vi "VEL.vi"(0 "System no.":i32=1 min=1 max=4 step=1, 2 "Axes to set":string[](array[string]), 3 "Velocity values":dbl[](array[numeric]) format="%.6f", 4 "No.of digits":i16=4, 5 "error in":errorcluster, 6 "Without axis ID?":bool) -> (14 "Controller error":bool, 19 "error out":errorcluster)   [LabVIEW 2026]
doc: "Sets velocity and checks for error. If Without axis ID? is TRUE, then Axes to set is ignored and first field of Velocity values array is used for velocity command. The velocity should not be set to 0. Number of digits is the number of digits after the decimal point in the velocity value(s) that will be sent. Controller error is TRUE if selected system reports an error code which is not 0.\n\nAnalog: Without axis ID? = FALSE; Velocity unit is µm/sec\n\nC-413: Without axis ID? = FALSE. Velocity unit is mm/s. Velocity settings made with VEL are present in RAM only and will be reset to default (parameter 0x06010400) when the controller is powered down or rebooted.\n\nC-867, C-877, C-884, C-891, Hydra, Pollux, Mercury_GCS: Without axis ID? = FALSE. Velocity unit is mm/s. The VEL command saves the parameters in RAM only. To save the currently valid parameters to flash ROM, where they become the power-on defaults, you must run WPA.vi. Parameter changes not saved with WPA will be lost when the controller is powered off.\n\nC-880: Without axis ID? = FALSE, for NanoCube axes command is not valid\n\nC-880K005: VI only supported when called through PI_Multix.vi\n\nC-885: Without axis ID? = FALSE. The VEL command saves the parameters in RAM only. For how to save the currently valid parameters to flash ROM, where they become the power-on defaults, please refer to the controller's user manual.\n\nE-516: Without axis ID? = FALSE. Velocity unit is µm/s. The VEL command saves the parameters in RAM only. To save the currently valid parameters to flash ROM, where they become the power-on defaults, you must run WPA.vi. Parameter changes not saved with WPA will be lost when the E-516 is powered off.\n\nE -517, E-518: Without axis ID? = FALSE. Velocity unit is µm/s in closed-loop operation and V/s in open-loop operation. Velocity settings made with VEL are present in RAM only and will be reset to default (\"Servo Loop Slew Rate\" value) when the controller is powered down or rebooted.\n\nE-709, E-712, E-725, E-727, E-753, E-754, E-861: Without axis ID? = FALSE. Velocity unit is µm/s. Velocity settings made with VEL are present in RAM only and will be reset to default (\"Servo Loop Slew Rate\" value) when the controller is powered down or rebooted.\n\nE-710: Without axis ID? = FALSE. Velocity unit is µm/ms.\n\nE-755: Without axis ID? = FALSE. Velocity unit is µm/s. Command not available for E-755.101.\n\nE-761: Without axis ID? = FALSE. Velocity unit is µm/ms.The VEL command saves the \"Servo Loop Slew Rate\" parameter in RAM only. To save the currently valid parameter to flash ROM, where it becomes the power-on defaults, you must run WPA.vi. Parameter changes not saved with WPA will be lost when the PC is powered off or the E-761 is rebooted.\n\nE-861: Without axis ID? = FALSE. The VEL setting only takes effect when the given axis is in closed-loop operation (servo on). For open-loop operation, use OVL instead. The maximum value which can be set with the VEL command is given by the Closed-loop velocity parameter, ID 0xA (can be changed with SPA and SEP). On power-on, the current closed-loop velocity is half the maximum.\n\nE-873, E-874: Without axis ID? = FALSE. The VEL command saves the parameters in RAM only. To save the currently valid parameters to flash ROM, where they become the power-on defaults, you must run WPA.vi. Parameter changes not saved with WPA will be lost when the controller is powered off.\n\nC-886: VEL command is only valid for velocity of additional axes. To set velocity of the parallel kinematics, please use the VLS command instead.\n\nC-887, F-206, M-8X0: For GCS syntax version = GCS 2.0 or higher (Check with CSV?.vi. If CSV?.vi is not supported, syntax version is GCS 1.0), VEL command is only valid for velocity of axes A and/or B, Without axis ID? = False. For platform velocity, VI sends command VLS instead, in this case Without axis ID? = TRUE. For axes K, L, M command is not valid.\nFor GCS syntax version = GCS 1.0, to set platform velocity: Without axis ID? = TRUE; to set velocity of axes A and/or B: Without axis ID? = False; axes K, L, M: command not valid. \n\nAll other systems: Without axis ID? = FALSE"
uses:
  Controller names.ctl
  Communication/Syntax.ctl
  Communication/Global1.vi
  Global2 (Array).vi
panel:
  # "Sets velocity and checks for error.  If \"Without axis ID\" is TRUE, \nthen \"Axes to set\" is ignored and first field of \"Velocity values\" \narray is used for velocity command by sending VEL for GCS 1.0 \nand VLS for GCS 2.0 or higher."
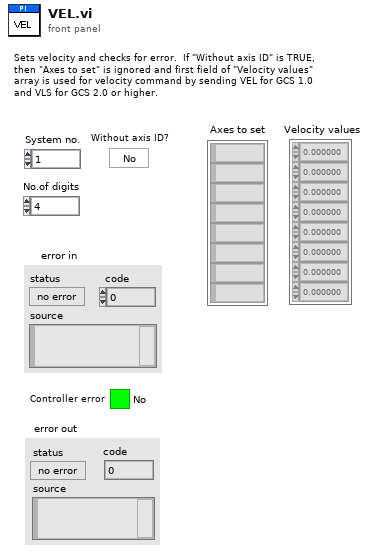
[diagram p1: front panel]
types:
  T1 = typedef "Syntax.ctl" = enum16{"GCS 1.0", "GCS 2.0", "GCS 3.0"}
  T2 = enum16{"Disable error check", "Force error check", "Use global settings"}
  T3 = typedef "Controller names.ctl" = enum16{"None", "Analog", "C-702", "C-413", "C-414", "C-843", "C-843.PM", "C-844", "C-848", "C-865", "C-866", "C-867", "C-877", "C-880", "C-884", "C-885", "C-886", "C-887", "C-891", "E-135", "E-516", "E-517", "E-518", "E-709", "E-710", "E-712", "E-725", "E-727", "E-753", "E-754", "E-755", "E-761", "E-816", "E-861", "E-870", "E-871", "E-872", "E-873", "E-874", "F-206", "HydraPollux", "M-840", "M-850", "M-8X0", "Mercury", "Mercury_GCS", "PI_GCS2"}
  T4 = cluster{"Conn. axes":string[], "Controller name":T3}[]
  T5 = cluster{"Conn. axes":string[], "Controller name":T3}
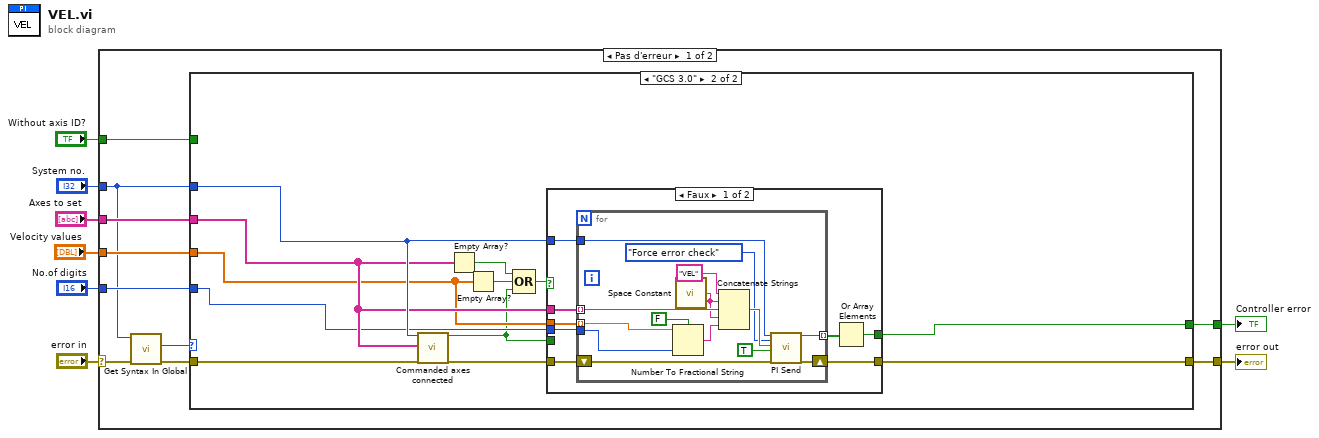
[diagram p0: block diagram]
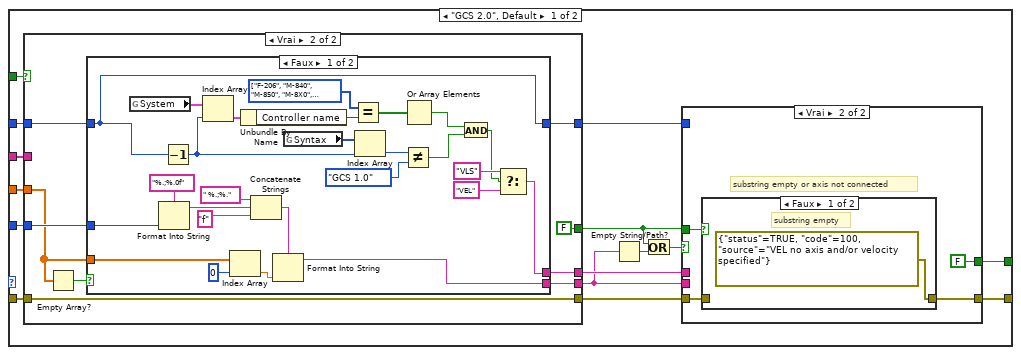
[diagram p2: hidden frame]
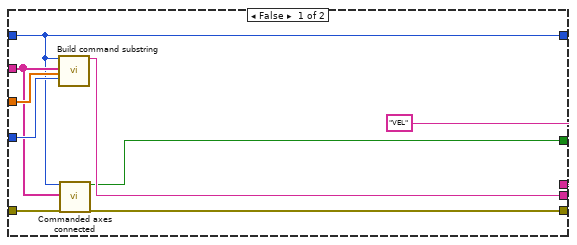
[diagram p3: hidden frame]
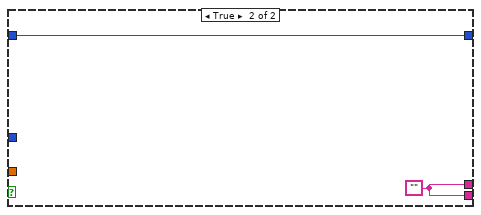
[diagram p4: hidden frame]
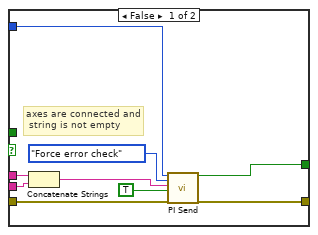
[diagram p5: hidden frame]
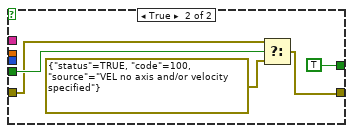
[diagram p7: hidden frame]
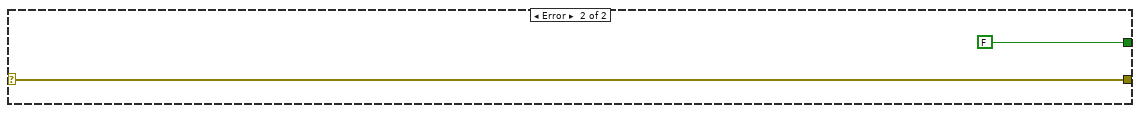
[diagram p8: hidden frame]
diagram:
  n1 = case shown="Pas d'erreur" "error in" {
    selector: "error in" -> [w11 w135]
    tunnel: [w18 w135] -> w8
    tunnel: "Velocity values" -> [w17 _]
    tunnel: "No.of digits" -> [w16 _]
    tunnel: "System no." -> [w9 _]
    tunnel: "Axes to set" -> [w15 _]
    tunnel: "Without axis ID?" -> [w14 _]
    tunnel: [w13 FALSE ("Controller error")] -> w1
    frame No Error {
      n2 = call "Get Syntax In Global.vi"("error in"=w11, "System no."=w9) -> ("error out"=w10:errorcluster, "Syntax"=w12:T1)  [unwired: 8 in]
      n3 = case shown="\"GCS 3.0\"" w12 {
        tunnel: [w33 w105] -> w18
        tunnel: w17 -> [w32 w101]
        tunnel: w16 -> [w31 w100]
        tunnel: w15 -> [w29 w102]
        tunnel: w14 -> [w28 _]
        tunnel: w9 -> [w27 w103]
        tunnel: w10 -> [w25 w104]
        tunnel: [w19 w96] -> w13
        frame "GCS 2.0", Default {
          n4 = case shown="Vrai" w28 {
            tunnel: [w42 w49] -> w24
            tunnel: w32 -> [w41 w46]
            tunnel: w31 -> [w40 w48]
            tunnel: w25 -> [w39 w51]
            tunnel: [w38 w51] -> w30
            tunnel: w29 -> [w37 _]
            tunnel: [w36 FALSE] -> w22
            tunnel: w27 -> [w34 w44]
            tunnel: ["VEL" w47] -> w26
            tunnel: [w34 w43] -> w20
            frame False {
              n5 = call "Build command substring.vi"("System no."=w34, "Affected axes"=w37, "Parameters"=w41, "No. of digits"=w40) -> ("Command substring"=w42:string)  [unwired: 3 in, 12 out]
              n6 = call "Commanded axes connected.vi"("System no."=w34, "Commanded axes"=w37, "error in"=w39) -> ("Controller error"=w36:bool, "error out"=w38:errorcluster)  [unwired: 1 in, 14 out]
            }
            frame True {
              n7 = Empty Array?(array=w46) -> (empty?=w45:bool)
              n8 = case shown="Faux" w45 {
                tunnel: [w77 w79] -> w49
                tunnel: w48 -> [w72 _]
                tunnel: w46 -> [w70 _]
                tunnel: [w56 w79] -> w47
                tunnel: w44 -> [w52 w78]
                tunnel: [w52 w78] -> w43
                frame False {
                  w66 = T3[] [enum."F-206", enum."M-840", enum."M-850", enum."M-8X0", enum."C-887"] items=["None", "Analog", "C-702", "C-413", "C-414", "C-843", "C-843.PM", "C-844", "C-848", "C-865", "C-866", "C-867", "C-877", "C-880", "C-884", "C-885", "C-886", "C-887", "C-891", "E-135", "E-516", "E-517", "E-518", "E-709", "E-710", "E-712", "E-725", "E-727", "E-753", "E-754", "E-755", "E-761", "E-816", "E-861", "E-870", "E-871", "E-872", "E-873", "E-874", "F-206", "HydraPollux", "M-840", "M-850", "M-8X0", "Mercury", "Mercury_GCS", "PI_GCS2"]
                  n9 = global read "Global2 (Array).vi" "System"() -> (w63:T4)
                  n10 = Format Into String(format string="%.;%.0f" ("Format String"), w72) -> (resulting string=w73:string)  [unwired: 2 in, 1 out]
                  n11 = Decrement(x=w52) -> (x-1=w60:i32)
                  n12 = Index Array(array=w63, index=w60) -> (element=w64:T5)
                  n13 = Index Array(array=w70, index=0 ("Index")) -> (element=w53:dbl)
                  n14 = Unbundle By Name(w64) -> ("Controller name"=w65:T3)
                  n15 = Concatenate Strings(" %.;%." ("Format String"), w73, "f" ("Format String")) -> (w71:string)
                  n16 = Format Into String(format string=w71, w53) -> (resulting string=w77:string)  [unwired: 2 in, 1 out]
                  n17 = global read "Global1.vi" "Syntax"() -> (w69:T1[])
                  n18 = Equal?(x=w66, y=w65) -> (x = y?=w67:bool[])
                  n19 = Index Array(array=w69, index=w60) -> (element=w68:T1)
                  n20 = Not Equal?(x=w68, y=Syntax."GCS 1.0") -> (x != y?=w62:bool)
                  n21 = Or Array Elements(Boolean array=w67) -> (logical OR=w61:bool)
                  n22 = And(x=w61, y=w62) -> (x .and. y?=w55:bool)
                  n23 = Select(t="VLS", s=w55, f="VEL") -> (s? t:f=w56:string)
                }
                frame True {
                  w79 = ""
                }
              }
            }
          }
          n24 = Empty String/Path?(string/path=w24) -> (empty?=w23:bool)
          n25 = Or(x=w22, y=w23) -> (x .or. y?=w21:bool)
          n26 = case shown="Vrai" w21 {
            tunnel: w24 -> [w88 _]
            tunnel: [w82 w92] -> w33
            tunnel: w30 -> [w85 w90]
            tunnel: w22 -> [_ w91]
            tunnel: w26 -> [w84 _]
            tunnel: w20 -> [w81 _]
            tunnel: [w80 FALSE ("Controller error")] -> w19
            frame False {
              # "axes are connected and\n string is not empty"
              n27 = Concatenate Strings(w84, w88) -> (w86:string)
              n28 = call "PI Send.vi"("System no."=w81, "Error check settings"=T2."Force error check", "String to send"=w86, "Attach termination char.?"=TRUE ("Attach Linefeed?"), "error in"=w85) -> ("Controller error"=w80:bool, "error out"=w82:errorcluster)  [unwired: 1 in, 12 out]
            }
            frame True {
              # "substring empty or axis not connected"
              n29 = case shown="Faux" w91 {
                tunnel: [errorcluster {"status"=TRUE, "code"=100, "source"="VEL no axis and/or velocity specified"} ("error out") w94] -> w92
                tunnel: w90 -> [_ w94]
                frame False {
                  # "substring empty"
                }
                frame True {
                  # "commanded axis not connected"
                }
              }
            }
          }
        }
        frame "GCS 3.0" {
          n30 = call "Commanded axes connected.vi"("System no."=w103, "Commanded axes"=w102, "error in"=w104) -> ("Controller error"=w95:bool, "error out"=w106:errorcluster)  [unwired: 15 out]
          n31 = Empty Array?(array=w102) -> (empty?=w99:bool)
          n32 = Empty Array?(array=w101) -> (empty?=w98:bool)
          n33 = Compound Arithmetic op=OR(w99, w98, w95) -> (w97:bool)
          n34 = case shown="Faux" w97 {
            tunnel: w106 -> [w114 w130]
            tunnel: [w113 w129] -> w105
            tunnel: w102 -> [w112 _]
            tunnel: w103 -> [w111 _]
            tunnel: w101 -> [w110 _]
            tunnel: w100 -> [w109 _]
            tunnel: [w107 TRUE] -> w96
            tunnel: w95 -> [_ w131]
            frame False {
              n35 = for {
                shift-right: [w128] -> w113
                shift-left: w114 -> [w127]
                tunnel: w112 -> [w123] mode=indexing
                tunnel: w110 -> [w120] mode=indexing
                tunnel: w111 -> [w121]
                tunnel: w109 -> [w118]
                tunnel: [w116] -> w108 mode=indexing
                n36 = Number To Fractional String(use system decimal point (T)=FALSE, number=w120, precision (6)=w118) -> (F-format string=w119:string)  [unwired: 1 in]
                n37 = call <vilib>:"Space Constant.vi"() -> ("String"=w122:string)
                n38 = Concatenate Strings("VEL", w122, w123, w122, w119) -> (w124:string)
                n39 = call "PI Send.vi"("System no."=w121, "Error check settings"=T2."Force error check", "String to send"=w124, "Attach termination char.?"=TRUE ("Attach Linefeed?"), "error in"=w127) -> ("Controller error"=w116:bool, "error out"=w128:errorcluster)  [unwired: 1 in, 12 out]
              }
              n40 = Or Array Elements(Boolean array=w108) -> (logical OR=w107:bool)
            }
            frame True {
              n41 = Select(t=w130, s=w131, f=errorcluster {"status"=TRUE, "code"=100, "source"="VEL no axis and/or velocity specified"} ("error out")) -> (s? t:f=w129:errorcluster)
            }
          }
        }
      }
    }
    frame Error {
    }
  }
  "error out" <- w8
  "Controller error" <- w1
